vi "isFactor function for kittens.vi"(10 "Numerator":dbl) -> ()   [LabVIEW 2012]
panel:
  out "isFactor":bool
  in  "Denominator":dbl
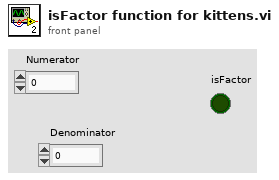
[diagram p1: front panel]
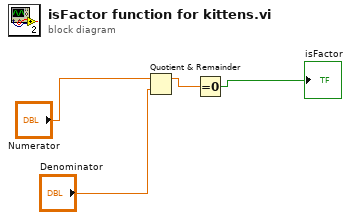
[diagram p0: block diagram]
diagram:
  n1 = Quotient & Remainder(x="Numerator", y="Denominator") -> (x-y*floor(x/y)=w2:dbl)  [unwired: 1 out]
  n2 = Equal To 0?(x=w2) -> (x = 0?=→"isFactor":bool)
